vi "Simulação.vi"() -> ()   [LabVIEW 2016]
panel:
  out "3D Picture":refnum<vi>(3d-picture)
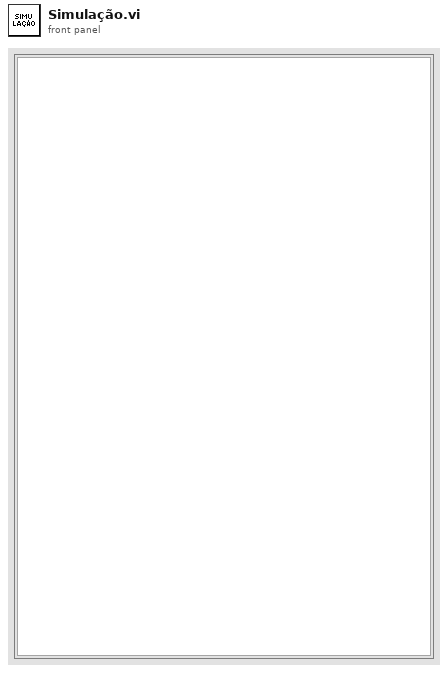
[diagram p1: front panel]
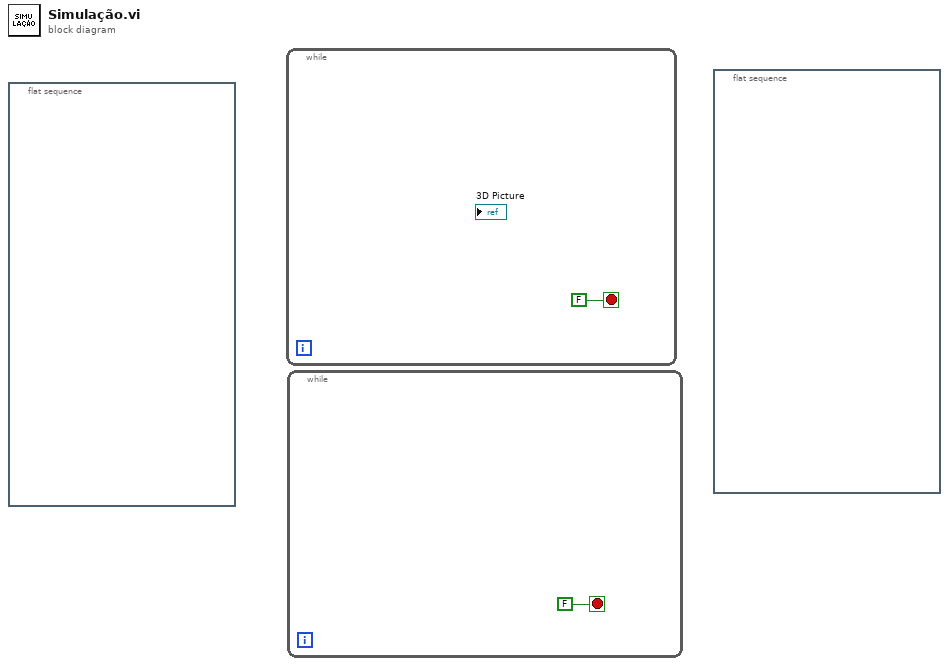
[diagram p0: block diagram]
diagram:
  n1 = flat-sequence {
    frame #0 {
    }
  }
  n2 = while {
    stop <- FALSE stop-if-true
  }
  n3 = while {
    stop <- FALSE stop-if-true
  }
  n4 = flat-sequence {
    frame #0 {
    }
  }
